vi "Iterative Write.vi"(5 "Username":string, 6 "Password":string, 7 "Address":string, 8 "Error In":errorcluster) -> (0 "Error Out":errorcluster)   [LabVIEW 2018, in "Tests.lvlib" / "SFTP File.lvlib"]
uses:
  SFTP File.lvlib
  <vilib>/addons/_JKI Toolkits/Caraya/classes/Test/Test.lvclass
  <vilib>/addons/_JKI Toolkits/Caraya/classes/Assert/Assert.lvclass
  src/Toolkit/SFTP File/SFTP File.lvclass
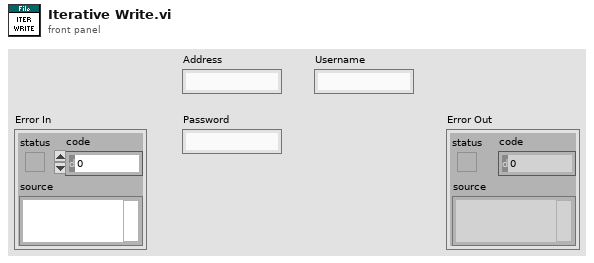
[diagram p1: front panel]
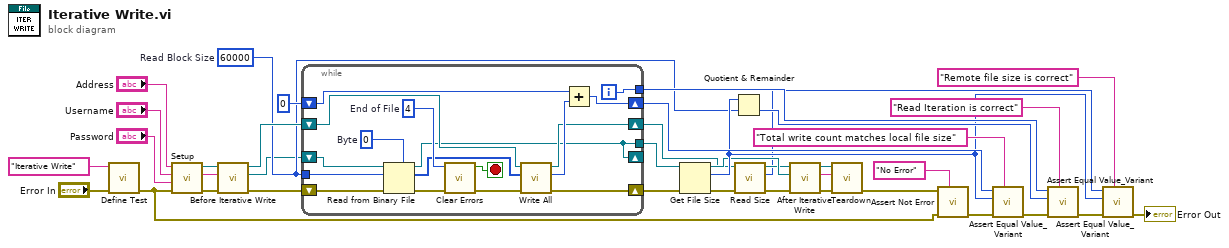
[diagram p0: block diagram]
diagram:
  w11 = i64 60000  # Read Block Size
  n1 = call <vilib>:"Define Test.vi"("error in (no error)"="Error In", "Label (VI Title)"="Iterative Write") -> ("error out"=w25:errorcluster)  [unwired: 9 in]
  n2 = call "Setup.vi"("Error In"=w25, "Password"="Password", "Username"="Username", "Address"="Address") -> ("Error Out"=w33:errorcluster, "Temporary File"=w29:string, "SFTP"=w35:refnum<class "SFTP.lvclass">)  [unwired: 5 in]
  n3 = call "Before Iterative Write.vi"("Error In"=w33, "Temporary File"=w29, "SFTP"=w35) -> ("Error Out"=w9:errorcluster, "Local"=w10:refnum<file>, "SFTP File"=w34:refnum<class "SFTP File.lvclass">)  [unwired: 6 in]
  n4 = while {
    tunnel: w11 -> [w47]
    shift-right: [w40] -> _
    shift-left: w10 -> [w55]
    shift-right: [w39] -> w6
    shift-left: w9 -> [w54]
    shift-right: [w48] -> w21
    shift-left: i64 0 -> [w51]
    tunnel: [w49] -> w17
    shift-right: [w43] -> w5
    shift-left: w34 -> [w42]
    tunnel: [w40] -> w8
    i -> [w49]
    stop <- w46 stop-if-true
    w50 = u8 0  # Byte
    w52 = 4  # End of File
    n5 = Read from Binary File(5:w50, 8:w54, 10:w47, 11:w55) -> (0:w53:errorcluster, 2:w41:u8[], 3:w40:refnum<file>)  [unwired: 2 in, 1 out]
    n6 = call <vilib>:"Clear Errors.vi"("error in (no error)"=w53, "specific error code to clear (0: all)"=w52) -> ("error out"=w45:errorcluster, "specific error cleared?"=w46:bool)  [unwired: 4 in]
    n7 = call "Write All.vi"("Error In"=w45, "Bytes"=w41, "SFTP File In"=w42) -> ("Error Out"=w39:errorcluster, "Block Write Count"=w44:i64, "SFTP File Out"=w43:refnum<class "SFTP File.lvclass">)  [unwired: 6 in]
    n8 = Add(x=w51, y=w44) -> (x+y=w48:i64)
  }
  n9 = Get File Size(file=w8, error in=w6) -> (refnum out=w7:refnum<file>, size (in bytes)=w12:i64, 0:w1:errorcluster)
  n10 = Quotient & Remainder(x=w12, y=w11) -> (floor(x/y)=w16:i64)  [unwired: 1 out]
  n11 = call "Read Size.vi"("Error In"=w1, "SFTP File In"=w5) -> ("Error Out"=w3:errorcluster, "File Size"=w2:u64, "SFTP File Out"=w4:refnum<class "SFTP File.lvclass">)  [unwired: 7 in]
  n12 = call "After Iterative Write.vi"("Error In"=w3, "Local"=w7, "SFTP File"=w4) -> ("Error Out"=w30:errorcluster, "Remote Path"=w32:string, "SFTP"=w31:refnum<class "SFTP.lvclass">)  [unwired: 6 in]
  n13 = call "Teardown.vi"("Error In"=w30, "Temporary File"=w32, "SFTP"=w31) -> ("Error Out"=w26:errorcluster)  [unwired: 8 in]
  n14 = call <vilib>:"Assert Not Error.vi"("Label"="No Error", "error in (no error)"=w25, "Not Error?"=w26) -> ("error out"=w23:errorcluster)  [unwired: 8 in]
  n15 = call <vilib>:"Assert Equal Value_Variant.vi"("Label"="Total write count matches local file size", "error in (no error)"=w23, "Y"=w12, "X"=w21) -> ("error out"=w19:errorcluster)  [unwired: 7 in]
  n16 = call <vilib>:"Assert Equal Value_Variant.vi"("Label"="Read Iteration is correct", "error in (no error)"=w19, "Y"=w16, "X"=w17) -> ("error out"=w15:errorcluster)  [unwired: 7 in]
  n17 = call <vilib>:"Assert Equal Value_Variant.vi"("Label"="Remote file size is correct", "error in (no error)"=w15, "Y"=w12, "X"=w2) -> ("error out"=→"Error Out":errorcluster)  [unwired: 7 in]
